vi "solar_write VoyagerExport.vi"(8 "error in (no error)":errorcluster, 10 "COSMOS Root":path, 11 "solar in":refnum<class "solar.lvclass">) -> (0 "error out":errorcluster, 3 "solar out":refnum<class "solar.lvclass">)   [LabVIEW 2018, in "solar.lvclass"]
doc: "This exports the Voyager interfaces and targets to the COSMOS directoy. If COSMOS Root is empty, this uses the built in COSMOS Root folder set by the SOLAR application.\nNote: Only call this function after all the target's packets are registered."
uses:
  solar.lvclass
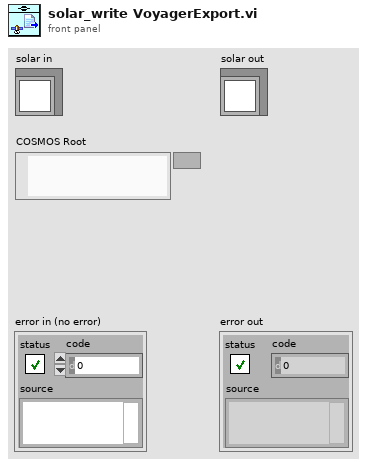
[diagram p1: front panel]
types:
  T1 = typedef "solar_voy_ctl Voyager Refnum.ctl" = refnum<k1>
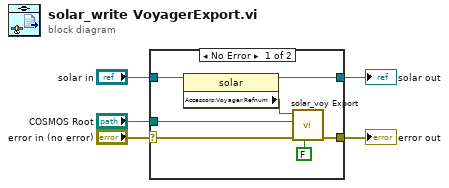
[diagram p0: block diagram]
diagram:
  n1 = case shown="No Error" "error in (no error)" {
    selector: "error in (no error)" -> [w7 w14]
    tunnel: "solar in" -> [w12 w13]
    tunnel: [w11 w13] -> w4
    tunnel: [w10 w14] -> w3
    tunnel: "COSMOS Root" -> [w8 _]
    frame No Error {
      n2 = property class="solar"(reference=w12) -> (reference out=w11:refnum<class "solar.lvclass">, "Accessors:Voyager.Refnum"=w9:T1)  [unwired: 1 in, 1 out]
      n3 = call "solar_voy Export.vi"("Suppress Errors? (T)"=FALSE, "error in (no error)"=w7, "COSMOS Root (\"\" = Use Default)"=w8, "Voyager Refnum in"=w9) -> ("error out"=w10:errorcluster)  [unwired: 6 in, 1 out]
    }
    frame Error {
    }
  }
  "error out" <- w3
  "solar out" <- w4
